vi "PlaceBallTactic.vi"(7 "firstCall":bool, 8 "error in (no error)":errorcluster, 9 "Game in":refnum<class "Game.lvclass">, 10 "Robot":refnum<class "Robot.lvclass">, 11 "PlaceBallTactic in":refnum<class "PlaceBallTactic.lvclass">) -> (0 "error out":errorcluster, 2 "Robot out":refnum<class "Robot.lvclass">, 3 "PlaceBallTactic out":refnum<class "PlaceBallTactic.lvclass">)   [LabVIEW 2020, in "PlaceBallTactic.lvclass"]
uses:
  PlaceBallTactic.lvclass
  C:/RoboIME/SSL_AI/Tactic_class/Tactic.lvclass
  Robot_class/Robot.lvclass
  Game_class/Game.lvclass
  Robot_class/tactics.ctl
  StatesPlaceBallTactic.ctl
  Tactic_class/Tactic.lvclass/Tactic.ctl
  Skillbook_class/Skillbook.lvclass/Skillbook.ctl
  Robot_class/Robot.lvclass/Robot.ctl
  PlaceBallTactic.lvclass/PlaceBallTactic.ctl
  Skillbook_class/Read PlaceBallSkill.vi
  Skillbook_class/Read MoveAwayFromBallSkill.vi
  Tactic_class/Read Skillbook.vi
  Write States.vi
  Robot_class/Write tactic.vi
  Skillbook_class/Skillbook.lvclass
  PlaceBallSkill_class/PlaceBallSkill.lvclass
  MoveAwayFromBallSkill_class/MoveAwayFromBallSkill.lvclass
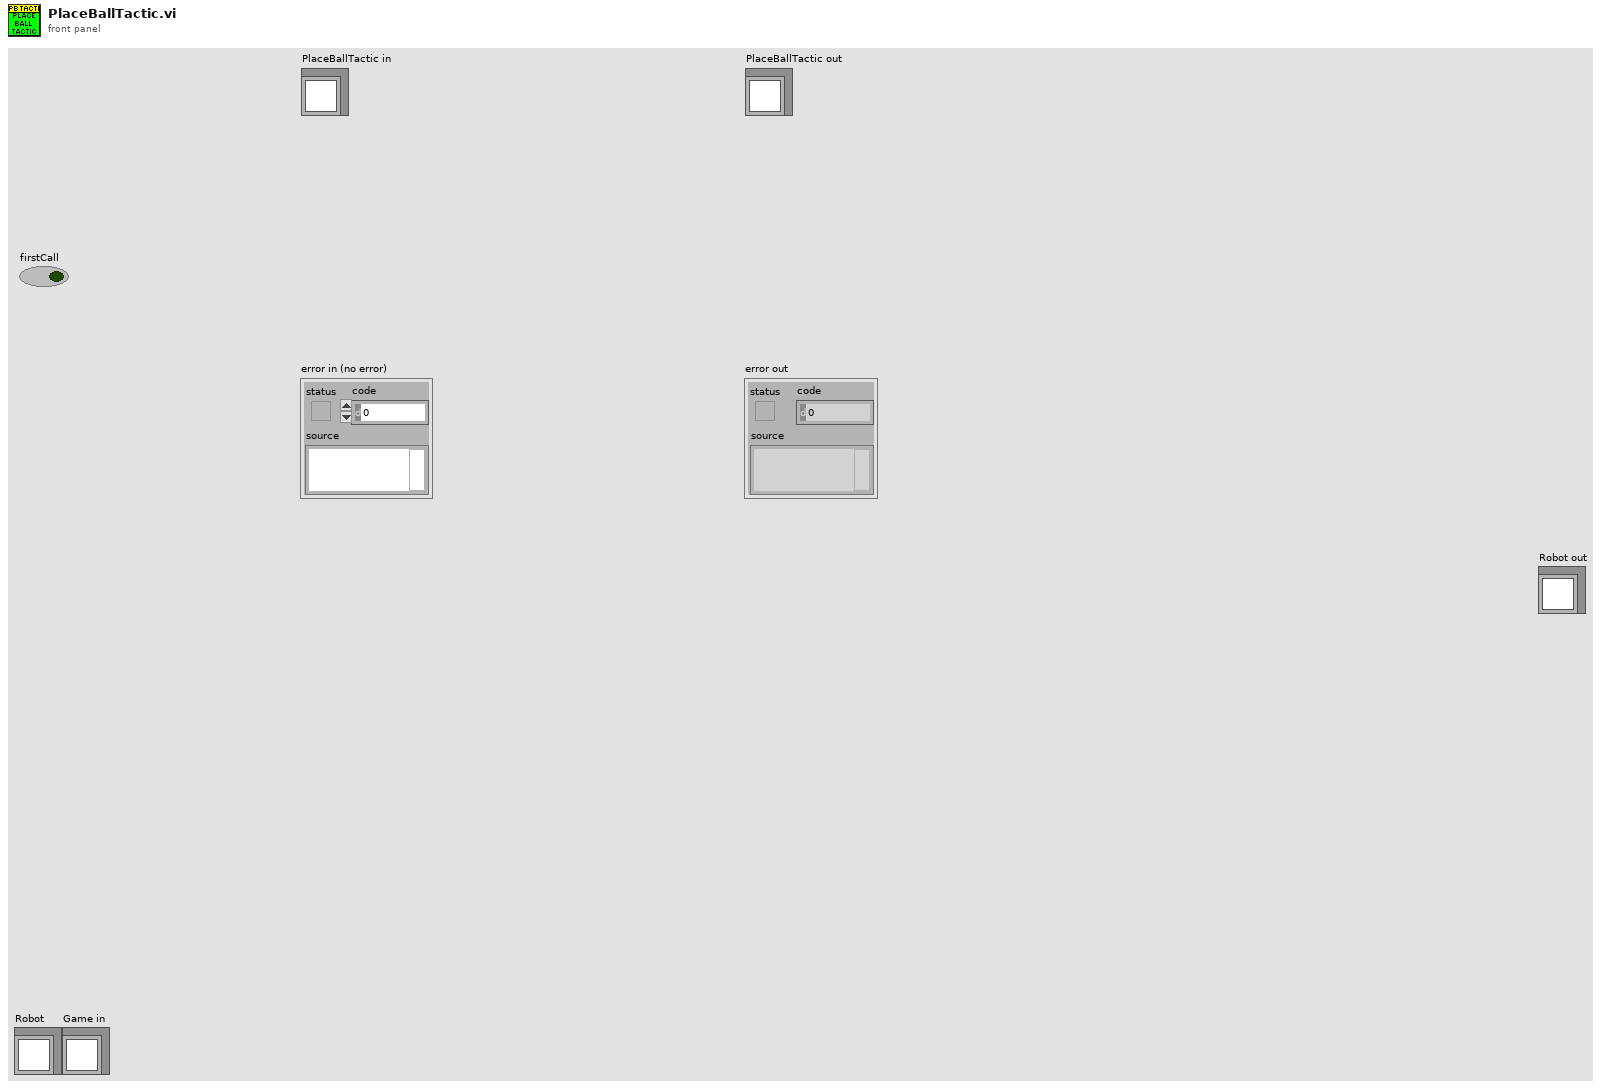
[diagram p1: front panel]
types:
  T1 = typedef "StatesPlaceBallTactic.ctl" = enum16{"PlaceBall", "Exit"}
  T2 = typedef "tactics.ctl" = enum16{"GoToBallPlacementPosition", "PlaceBall", "GoToBallPlacement", "5Robots", "BallPlacementEnemy", "ReceivePassInFuturePoint", "Roller", "PrepareRollToPassRollerGoTo", "PrepareRollToPassReceiverGoTo", "WaitRoll", "PositionToRoll", "PenaltyAttacker", "PassObserver", "PenaltyDefense", "TableReceiverTactic", "Test", "DefendGoal", "Marker", "FollowAttacker", "DefendArea", "Shoot", "AttackerAimGoal", "AttackerBallOutOfField", "AttackerBlock", "AttackerStop", "Duelist", "Halt", "ZigZag", "GoTo", "Timeout", "KickToBestRobot", "KickToPassReceiver", "PositionToReceivePass", "WaitPass"}
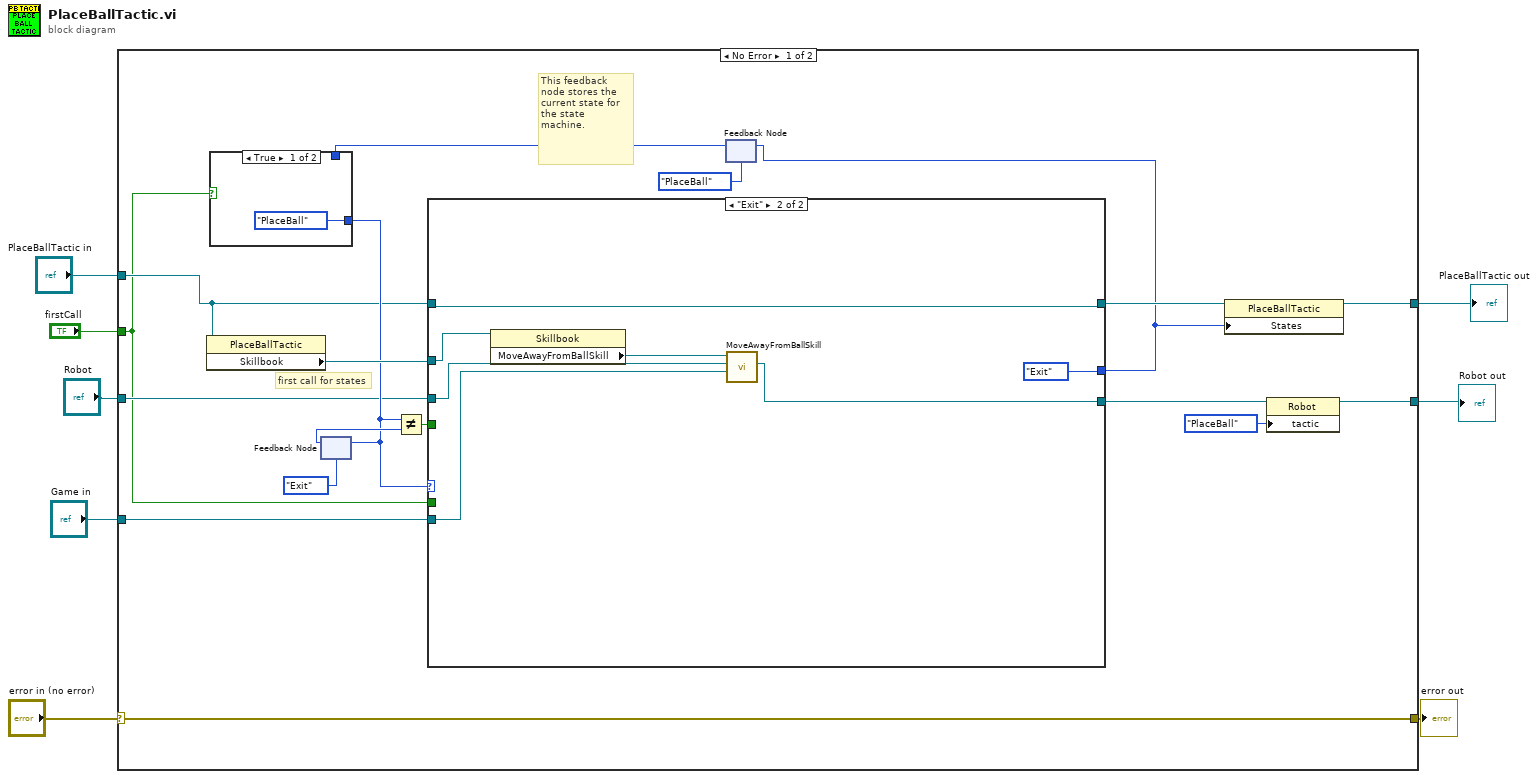
[diagram p0: block diagram]
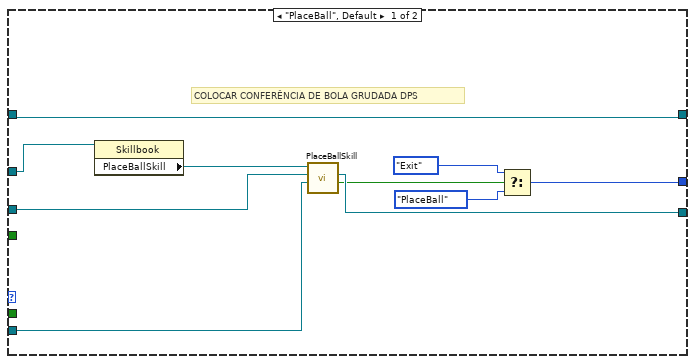
[diagram p3: hidden frame]
diagram:
  n1 = case shown="No Error" "error in (no error)" {
    selector: "error in (no error)" -> [w26 w47]
    tunnel: [w26 w47] -> w7
    tunnel: [w17 w46] -> w5
    tunnel: "PlaceBallTactic in" -> [w18 w46]
    tunnel: [w16 _] -> w1
    tunnel: "Robot" -> [w15 _]
    tunnel: "firstCall" -> [w14 _]
    tunnel: "Game in" -> [w10 _]
    frame No Error {
      # "first call for states"
      # "This feedback node stores the current state for the state machine."
      n2 = property class="PlaceBallTactic"(reference=w18) -> ("Skillbook"=w25:refnum<class "Skillbook.lvclass">)  [unwired: 1 in, 2 out]
      n3 = feedback #1(StatesPlaceBallTactic."Exit" ("States")) -> (w21:T1)
      n4 = feedback #2(StatesPlaceBallTactic."PlaceBall" ("States")) -> (w22:T1)
      n5 = case shown="True" w14 {
        tunnel: [StatesPlaceBallTactic."PlaceBall" ("States") w28] -> w20
        tunnel: w22 -> [_ w28]
        frame True {
        }
        frame False {
        }
      }
      n6 = feedback-in #1(w20) -> ()
      n7 = Not Equal?(x=w20, y=w21) -> (x != y?=w19:bool)
      n8 = case shown="\"Exit\"" w20 {
        tunnel: w25 -> [w37 w44]
        tunnel: w15 -> [w34 w40]
        tunnel: [w35 w41] -> w23
        tunnel: [w38 w45] -> w24
        tunnel: w18 -> [w38 w45]
        tunnel: w14 -> [_ _]
        tunnel: w19 -> [_ _]
        tunnel: [w30 StatesPlaceBallTactic."Exit" ("States")] -> w12
        tunnel: w10 -> [w29 w39]
        frame "PlaceBall", Default {
          # "COLOCAR CONFERÊNCIA DE BOLA GRUDADA DPS"
          n9 = property class="Skillbook"(reference=w37) -> ("PlaceBallSkill"=w36:refnum<class "PlaceBallSkill.lvclass">)  [unwired: 1 in, 2 out]
          n10 = call "PlaceBallSkill.vi"("Game"=w29, "Robot"=w34, "PlaceBallSkill in"=w36) -> ("finishedPlaceBall"=w33:bool, "Robot out"=w35:refnum<class "Robot.lvclass">)  [unwired: 5 in, 2 out]
          n11 = Select(t=StatesPlaceBallTactic."Exit" ("States"), s=w33, f=StatesPlaceBallTactic."PlaceBall" ("States")) -> (s? t:f=w30:T1)
        }
        frame "Exit" {
          n12 = property class="Skillbook"(reference=w44) -> ("MoveAwayFromBallSkill"=w42:refnum<class "MoveAwayFromBallSkill.lvclass">)  [unwired: 1 in, 2 out]
          n13 = call "MoveAwayFromBallSkill.vi"("Game in"=w39, "Robot"=w40, "MoveAwayFromBallSkill in"=w42) -> ("Robot out"=w41:refnum<class "Robot.lvclass">)  [unwired: 6 in, 2 out]
        }
      }
      n14 = feedback-in #2(w12) -> ()
      n15 = property class="PlaceBallTactic"(reference=w24, "States"=w12) -> (reference out=w17:refnum<class "PlaceBallTactic.lvclass">)  [unwired: 1 in, 1 out]
      n16 = property class="Robot"(reference=w23, "tactic"=tactics."PlaceBall") -> (reference out=w16:refnum<class "Robot.lvclass">)  [unwired: 1 in, 1 out]
    }
    frame Error {
    }
  }
  "error out" <- w7
  "PlaceBallTactic out" <- w5
  "Robot out" <- w1
